vi "GageTransferI8.vi"(4 "Length (4096)":dbl=4096.0, 5 "Start (0)":dbl, 6 "Segment (1)":u32=1, 7 "Mode (0)":u32 step=1, 8 "Channel (0)":u16 step=1, 9 "Handle Cluster":T1) -> (0 "Error Code":i32, 1 "Actual Length":dbl, 2 "Raw Data":i16[](array[numeric]), 3 "Actual Start":dbl)   [LabVIEW 2013]
doc: "This VI transfers the data from one channel of the CompuScope system identified by Handle Cluster, which is obtained by calling CsTool-GetSystem.vi. For accurate interpretation of the transferred data, the user should always use the returned Actual Start and Actual Length, and not the requested values. \n\nThis VI can be used for transferring data from 8, 12, 14, and 16 bit CompuScope hardware. Data are transferred from on-board CompuScope memory to PC RAM using PCI Bus Mastering at rates of up to 200 MB/s. \n\nInternally, CsTool-Transfer.vi converts the raw integer ADC code values into double variable voltage values. For more rapid data access, the user may remove the voltage conversion step. The VI will not return programmatic control to LabVIEW until all of the data have been transferred. \n\nIf the call is successful, a 1 is returned in the Error Code indicator. If the call is unsuccessful, an appropriate error code is returned. A descriptive error string may be obtained by calling CsTool-ErrorHandler.vi.\n\n\nInput Value Descriptions:\n\nChannel\nThis integer value specifies the channel from which data are to be transferred. The default value is 0 for the first channel in the CompuScope system. Channels in a LabVIEW CompuScope system begin at 0. If an invalid channel number is given, an error will be returned. Please see the CompuScope hardware manual for more information on channel enumeration.\n\nMode\nThis integer value determines the current transfer mode. Currently, the only valid value for this input is 0.\n\nSegment(1)\nThis integer value determines which Multiple Record segment is to be transferred, if the CompuScope hardware was operating in Multiple Record Mode. For Single Record Mode acquisitions, the user must always set the Record value to 1, which is the default value. If the Record value is too large, an error code will be returned. \n\nStart\nThis double variable value determines the requested starting point of the data transfer from CompuScope memory to PC RAM. Start is specified relative to the trigger address for the acquisition. A Start value of 0 will cause data transfer to begin at the trigger address. Negative Start values are used for the transfer of pre-trigger data. Positive Start values may be used to begin transfer after the trigger address. The default Start value is 0. \n\nLength\nThis double variable value specifies the amount of data, in samples, to be transferred. The default value is 4096. \n\nData in Volts\nThis array variable, of type double, is the LabVIEW buffer variable into which transferred data are returned. The size of the array will be at least Length samples. Data are returned as voltage values, whose conversion depends upon the resolution of the CompuScope system and on the current input range.\n\nActual Start\nThis double variable value returns the actual start point of the data array. The Actual Start may be lower than the requested Start value. This is because the CompuScope memory architecture may force the drivers to download data from an earlier point than the start position. For example, if Start is input to CsTool-Transfer.vi as 0, the Actual Start may return as -2, indicating that two extra samples were returned before the Start position. \n\nThe user must account for the discrepancy between the Start and the Actual Start. The user may choose to ignore samples transferred from before the Start position. Alternatively, the user may conserve these samples, accounting for the fact that the values begin at Actual Start. \n\nActual Length\nThis double variable value returns the actual amount of data transferred, which may be different from the requested Length. The difference, if any, results from CompuScope memory architecture."
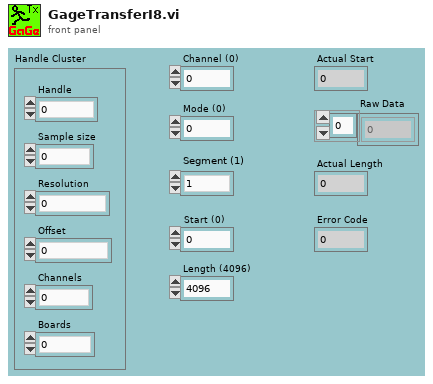
[diagram p1: front panel]
types:
  T1 = cluster{"Handle":u32, "Sample size":u32, "Resolution":i32, "Offset":i32, "Channels":u32, "Boards":u32}
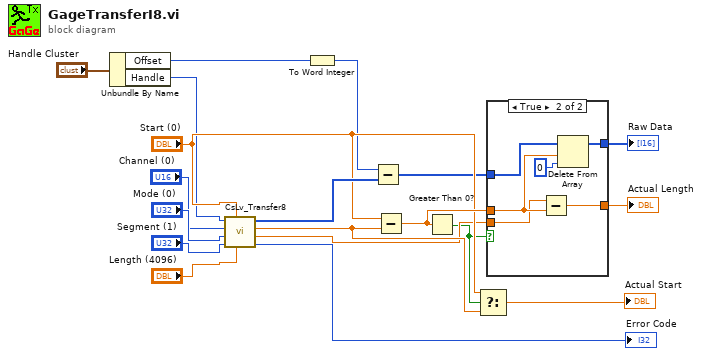
[diagram p0: block diagram]
diagram:
  n1 = Unbundle By Name("Handle Cluster") -> ("Offset"=w14:i32, "Handle"=w1:u32)
  n2 = call <instrlib>:"CsLv_Transfer8.vi"("Length (4096)"="Length (4096)", "Start (0)"="Start (0)", "Segment (1)"="Segment (1)", "Mode (0)"="Mode (0)", "Channel (0)"="Channel (0)", "Handle"=w1) -> ("Error Code"=→"Error Code":i32, "Actual Length"=w7:dbl, "Actual Start"=w8:dbl, "Buffer"=w15:u8[])
  n3 = To Word Integer(number=w14) -> (16bit integer=w2:i16)
  n4 = Subtract(x=w2, y=w15) -> (x-y=w3:i16[])
  n5 = Subtract(x="Start (0)", y=w8) -> (x-y=w12:dbl)
  n6 = Greater Than 0?(x=w12) -> (x > 0?=w6:bool)
  n7 = Select(t="Start (0)", s=w6, f=w8) -> (s? t:f=→"Actual Start":dbl)
  n8 = case shown="True" w6 {
    tunnel: w12 -> [_ w26]
    tunnel: w7 -> [w21 w25]
    tunnel: [w21 w24] -> w9
    tunnel: [w20 w23] -> w4
    tunnel: w3 -> [w20 w22]
    frame False {
    }
    frame True {
      n9 = Subtract(x=w25, y=w26) -> (x-y=w24:dbl)
      n10 = Delete From Array(array=w22, length=w26, index=0) -> (array with subset deleted=w23:i16[])  [unwired: 1 out]
    }
  }
  "Raw Data" <- w4
  "Actual Length" <- w9
